vi "read.vi"(8 "error in (no error)":errorcluster, 11 "SerialReal in":refnum<class "SerialReal.lvclass">) -> (0 "error out":errorcluster, 2 "stringRead":string, 3 "SerialReal out":refnum<class "SerialReal.lvclass">)   [LabVIEW 2015, in "SerialProtocols.lvlib" / "SerialReal.lvclass"]
uses:
  <userlib>/Common/SerialProtocols/SerialProtocol/SerialReal/SerialReal.lvclass
  <userlib>/Common/SerialProtocols/SerialProtocol/SerialReal/SerialReal.lvclass/SerialReal.ctl
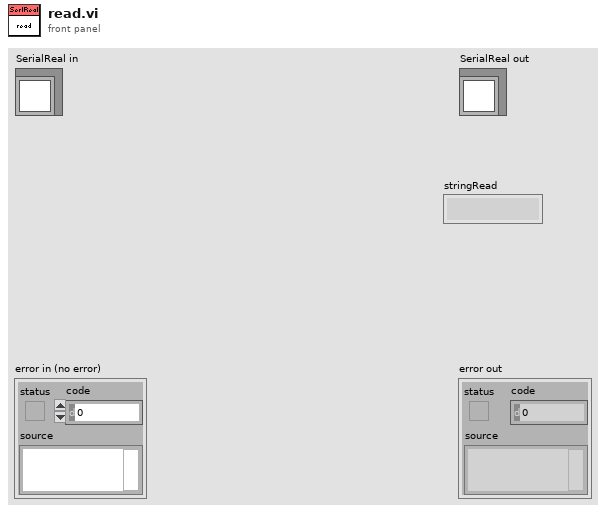
[diagram p1: front panel]
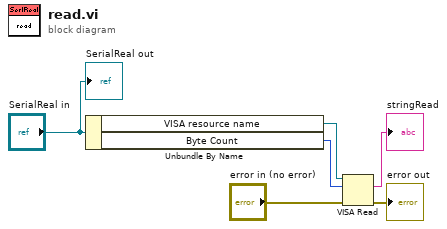
[diagram p0: block diagram]
diagram:
  n1 = Unbundle By Name("SerialReal in") -> ("VISA resource name"=w3:refnum<visa-resource-name>, "Byte Count"=w1:u32)
  n2 = VISA Read(VISA resource name=w3, byte count=w1, error in (no error)="error in (no error)") -> (read buffer=→"stringRead":string, error out=→"error out":errorcluster)  [unwired: 2 out]
  "SerialReal out" <- "SerialReal in"
